vi "Oven_PLC_Communication.vi"() -> ()   [LabVIEW 2017]
uses:
  <vilib>/NI/Modbus Library/API/Wrapper/Create TCP Master.vi
  <vilib>/NI/Modbus Library/API/master/Modbus Master.lvclass
  <vilib>/NI/Modbus Library/API/Wrapper/API Main.lvlib
panel:
  in  "stop 2":bool
  in  "number of register":u16=2
  in  "starting address":u16=60021
  in  "address":string="192.168.1.5"
  in  "error in":errorcluster
  in  "stop":bool
  out "register values":u16[](array[numeric])
  out "error out":errorcluster
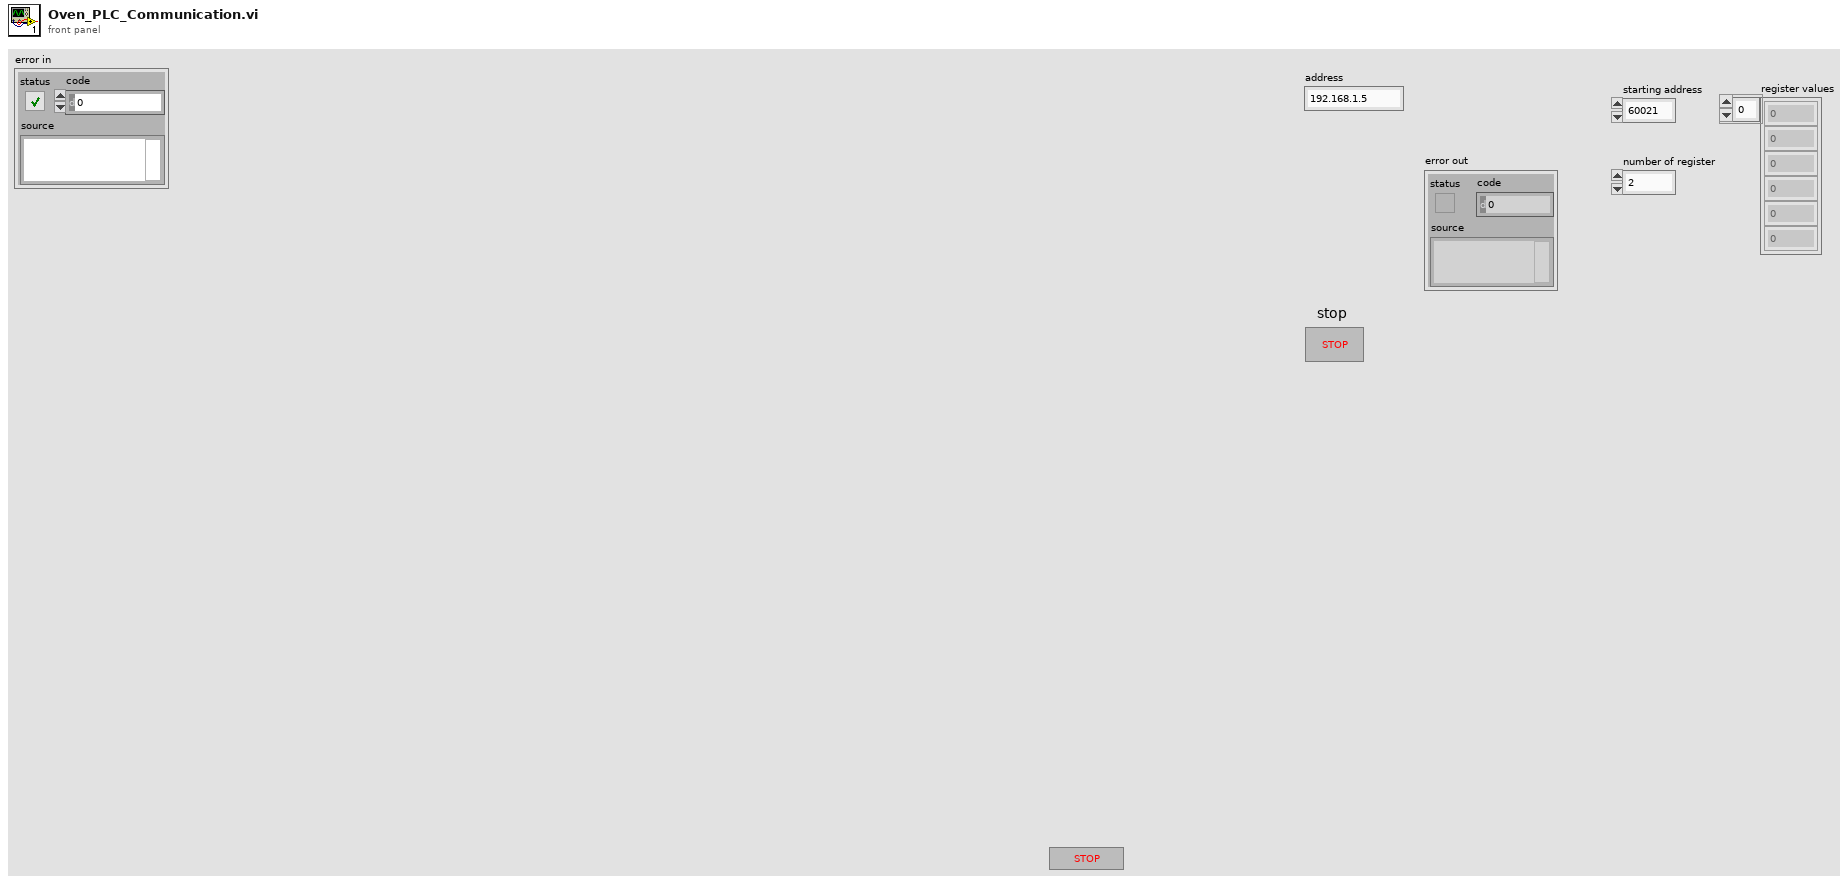
[diagram p1: front panel]
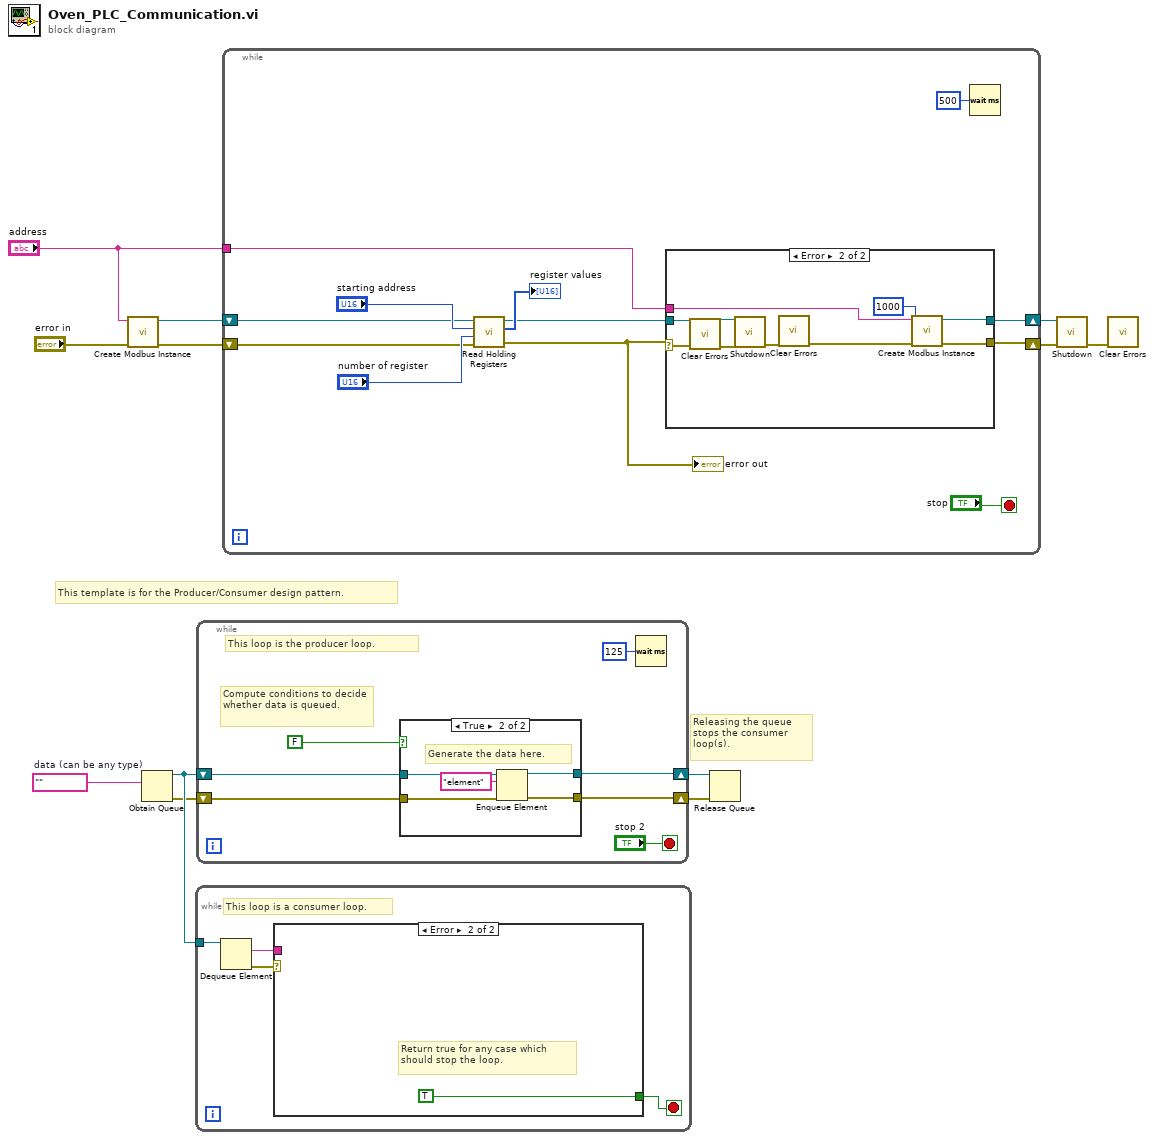
[diagram p0: block diagram]
diagram:
  w1 = ""  # data (can be any type)
  # "Releasing the queue stops the consumer loop(s)."
  # "This template is for the Producer/Consumer design pattern."
  n1 = call-poly <vilib>:"Create Modbus Instance.vi"("error in"="error in", "address"="address") -> ("error out"=w10:errorcluster, "TCP master instance"=w9:refnum<class "Modbus Master.lvclass">)  [unwired: 8 in]
  n2 = Obtain Queue(element data type=w1) -> (queue out=w5:refnum<queue>, error out=w4:errorcluster)  [unwired: 4 in, 1 out]
  n3 = while {
    tunnel: w5 -> [w16]
    stop <- w13 stop-if-true
    # "This loop is a consumer loop."
    n4 = Dequeue Element(queue=w16) -> (element=w14:string, error out=w15:errorcluster)  [unwired: 2 in, 2 out]
    n5 = case shown="Error" w15 {
      tunnel: w14 -> [_ _]
      tunnel: [_ TRUE] -> w13
      frame No Error {
        # "This is where you process the data obtained from the queue."
      }
      frame Error {
        # "Return true for any case which should stop the loop."
      }
    }
  }
  n6 = while {
    shift-right: [w20] -> w2
    shift-left: w4 -> [w21]
    shift-right: [w22] -> w3
    shift-left: w5 -> [w23]
    stop <- "stop 2" stop-if-true
    # "Compute conditions to decide whether data is queued."
    # "This loop is the producer loop."
    n7 = case shown="True" FALSE ("Case Constant\n(See Context Help)") {
      tunnel: w23 -> [w26 w31]
      tunnel: [w26 w30] -> w22
      tunnel: w21 -> [w25 w29]
      tunnel: [w25 w28] -> w20
      frame False {
      }
      frame True {
        # "Generate the data here."
        n8 = Enqueue Element(queue=w31, element="element", error in (no error)=w29) -> (queue out=w30:refnum<queue>, error out=w28:errorcluster)  [unwired: 1 in, 1 out]
      }
    }
    n9 = Wait (ms)(milliseconds to wait=u32 125) -> ()  [unwired: 1 out]
  }
  n10 = while {
    shift-right: [w43] -> w12
    shift-left: w9 -> [w38]
    shift-right: [w42] -> w11
    shift-left: w10 -> [w39]
    tunnel: "address" -> [w33]
    stop <- "stop" stop-if-true
    n11 = call-dynamic "Read Holding Registers.vi"("error in"=w39, "number of inputs"="number of register", "starting address"="starting address", "Modbus master in"=w38) -> ("error out"=w35:errorcluster, "register values"=→"register values":u16[], "Modbus master out"=w34:refnum<class "Modbus Master.lvclass">)  [unwired: 5 in]
    "error out" <- w35
    n12 = case shown="Error" w35 {
      selector: w35 -> [w44 w54]
      tunnel: w34 -> [w45 w52]
      tunnel: [w45 w49] -> w43
      tunnel: [w44 w48] -> w42
      tunnel: w33 -> [_ w46]
      frame No Error {
      }
      frame Error {
        n13 = call <vilib>:"Clear Errors.vi"("error in (no error)"=w54) -> ("error out"=w53:errorcluster)  [unwired: 5 in, 1 out]
        n14 = call-dynamic "Shutdown.vi"("error in"=w53, "Modbus master in"=w52) -> ("error out"=w51:errorcluster)  [unwired: 9 in]
        n15 = call <vilib>:"Clear Errors.vi"("error in (no error)"=w51) -> ("error out"=w50:errorcluster)  [unwired: 5 in, 1 out]
        n16 = call-poly <vilib>:"Create Modbus Instance.vi"("error in"=w50, "connect timeout ms"=1000, "address"=w46) -> ("error out"=w48:errorcluster, "TCP master instance"=w49:refnum<class "Modbus Master.lvclass">)  [unwired: 7 in]
      }
    }
    n17 = Wait (ms)(milliseconds to wait=u32 500) -> ()  [unwired: 1 out]
  }
  n18 = Release Queue(queue=w3, error in (no error)=w2) -> ()  [unwired: 1 in, 3 out]
  n19 = call-dynamic "Shutdown.vi"("error in"=w11, "Modbus master in"=w12) -> ("error out"=w7:errorcluster)  [unwired: 9 in]
  n20 = call <vilib>:"Clear Errors.vi"("error in (no error)"=w7) -> ()  [unwired: 5 in, 2 out]
